vi "msgsBuilder_MasterMessage.vi"(0 "msg in":string, 5 "statusString":string, 7 "liftState":i32, 9 "position":cluster{"x":dbl, "y":dbl, "z":dbl}, 11 "avgDist":sgl) -> (4 "msg out":string)   [LabVIEW 2016]
uses:
  <userlib>/ROS for LabVIEW Software/ROS/MessageBuilding/std_msgs/subs/stringScalar.vi
  <userlib>/ROS for LabVIEW Software/ROS/MessageBuilding/std_msgs/subs/i32Scalar.vi
  <userlib>/ROS for LabVIEW Software/ROS/MessageBuilding/std_msgs/subs/float32Scalar.vi
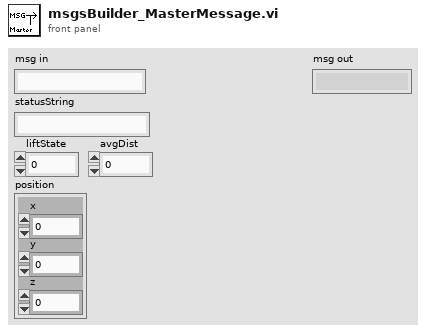
[diagram p1: front panel]
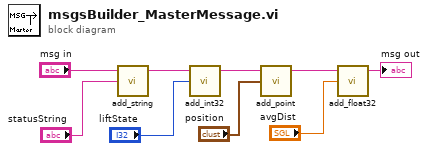
[diagram p0: block diagram]
diagram:
  n1 = call-poly <userlib>:"add_string.vi"("String"="statusString", "msg in"="msg in") -> ("msg out"=w7:string)  [unwired: 3 in]
  n2 = call-poly <userlib>:"add_int32.vi"("Numeric"="liftState", "msg in"=w7) -> ("msg out"=w5:string)  [unwired: 3 in]
  n3 = call <userlib>:"add_point.vi"("Point"="position", "msg in"=w5) -> ("msg out"=w3:string)  [unwired: 3 in]
  n4 = call-poly <userlib>:"add_float32.vi"("Numeric"="avgDist", "msg in"=w3) -> ("msg out"=→"msg out":string)  [unwired: 3 in]
